vi "Read States.vi"(8 "error in (no error)":errorcluster, 11 "AttackerAimGoalTactic in":refnum<class "AttackerAimGoalTactic.lvclass">) -> (0 "error out":errorcluster, 2 "States":T1, 3 "AttackerAimGoalTactic out":refnum<class "AttackerAimGoalTactic.lvclass">)   [LabVIEW 2018, in "AttackerAimGoalTactic.lvclass"]
uses:
  AttackerAimGoalTactic.lvclass
  States.ctl
  AttackerAimGoalTactic.lvclass/AttackerAimGoalTactic.ctl
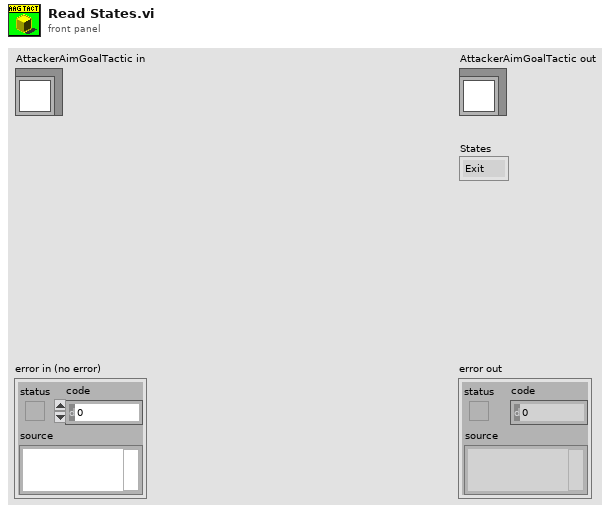
[diagram p1: front panel]
types:
  T1 = typedef "AttackerAimGoalTactic.lvclass/States.ctl" = enum16{"Exit", "AimGoal"}
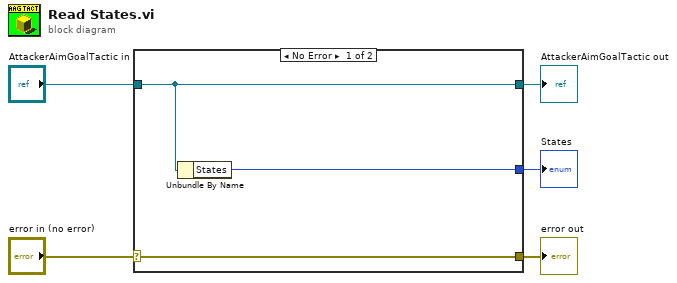
[diagram p0: block diagram]
diagram:
  n1 = case shown="No Error" "error in (no error)" {
    selector: "error in (no error)" -> [w8 w9]
    tunnel: [w8 w9] -> w4
    tunnel: [w7 w10] -> w2
    tunnel: "AttackerAimGoalTactic in" -> [w7 w10]
    tunnel: [w6 _] -> w1
    frame No Error {
      n2 = Unbundle By Name(w7) -> ("States"=w6:T1)
    }
    frame Error {
    }
  }
  "error out" <- w4
  "AttackerAimGoalTactic out" <- w2
  "States" <- w1
